vi "WPI_DigitalOutputOpen.vi"(8 "error in (no error)":errorcluster, 10 "DIO Channel":T1=enum."DIO 1") -> (0 "error out":errorcluster, 3 "DigitalOutputDevRef":T2={"DIO Channel"=enum."DIO 1", "DevStatus"={"status"=FALSE, "code"=0, "source"=""}})   [LabVIEW 2017]
doc: "Creates a reference to the digital output you specify. You must open a reference before using any other VIs on this palette.\n\nThis software is licensed. Open the labview\\readme\\WPI Robotics Library Open Source License.txt file for more information."
uses:
  <vilib>/Rock Robotics/WPI/DigitalOutput/WPI_DigitalOutputDevRef.ctl
  <vilib>/Rock Robotics/SystemInterfaces/DIO/FPGA_DIOChannel.ctl
  <vilib>/Rock Robotics/WPI/DigitalModule/WPI_DigitalModuleDIOCacheOp.ctl
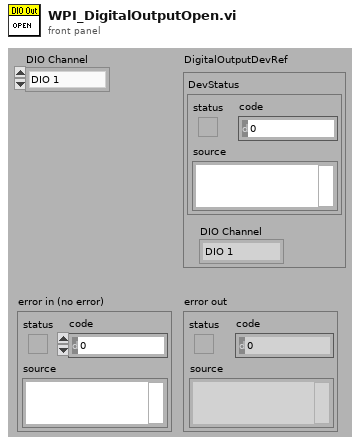
[diagram p1: front panel]
types:
  T1 = typedef "FPGA_DIOChannel.ctl" = enum8{"DIO 0", "DIO 1", "DIO 2", "DIO 3", "DIO 4", "DIO 5", "DIO 6", "DIO 7", "DIO 8", "DIO 9", "DIO MXP 0", "DIO MXP 1", "DIO MXP 2", "DIO MXP 3", "DIO MXP 4", "DIO MXP 5", "DIO MXP 6", "DIO MXP 7", "DIO MXP 8", "DIO MXP 9", "DIO MXP 10", "DIO MXP 11", "DIO MXP 12", "DIO MXP 13", "DIO MXP 14", "DIO MXP 15", "SPI Port CS1", "SPI Port CS2", "SPI Port CS3", "SPI Port MISO", "SPI Port MOSI", "Invalid"}
  T2 = typedef "WPI_DigitalOutputDevRef.ctl" = cluster{"DIO Channel":T1, "DevStatus":errorcluster}
  T3 = typedef "WPI_DigitalModuleDIOCacheOp.ctl" = enum16{"Acquire", "Release", "Status"}
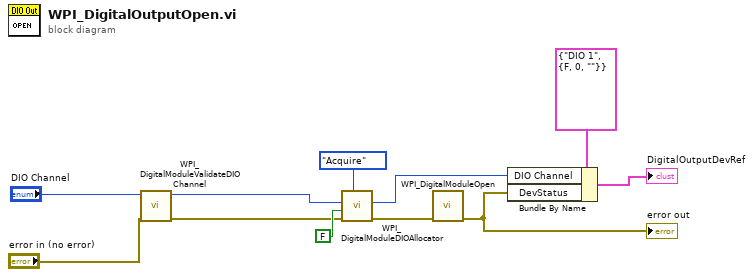
[diagram p0: block diagram]
diagram:
  n1 = call <vilib>:"WPI_DigitalModuleValidateDIOChannel.vi"("error in (no error)"="error in (no error)", "DIOChannel"="DIO Channel") -> ("error out"=w1:errorcluster, "DIOChannel"=w6:T1)  [unwired: 8 out]
  n2 = call <vilib>:"WPI_DigitalModuleDIOAllocator.vi"("AllocatedDIOMutex"=WPI_DigitalModuleDIOCacheOp."Acquire", "error in (no error)"=w1, "Input? (F)"=FALSE, "DIOChannel"=w6) -> ("error out"=w4:errorcluster, "Allocated DIOChannel"=w2:T1)  [unwired: 1 in, 5 out]
  n3 = call <vilib>:"WPI_DigitalModuleOpen.vi"("error in (no error)"=w4) -> ("error out"=w9:errorcluster)  [unwired: 1 in, 9 out]
  "error out" <- w9
  n4 = Bundle By Name(cluster=T2 {"DIO Channel"=enum."DIO 1", "DevStatus"={"status"=FALSE, "code"=0, "source"=""}} ("DigitalOutputDevRef"), "DIO Channel"=w2, "DevStatus"=w9) -> (→"DigitalOutputDevRef":T2)
